vi "Celsius To Kelvin.vi"(11 "Celsius":dbl) -> (3 "Kelvin":dbl)   [LabVIEW 2015]
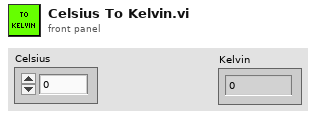
[diagram p1: front panel]
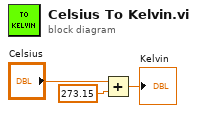
[diagram p0: block diagram]
diagram:
  n1 = Add(x="Celsius", y=273.15) -> (x+y=→"Kelvin":dbl)
